vi "testArea.vi"() -> ()   [LabVIEW 2019]
panel:
  out "output array":dbl[](array[numeric])
  out "Area":dbl
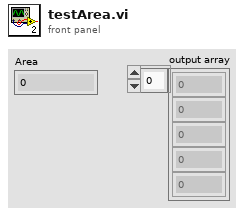
[diagram p1: front panel]
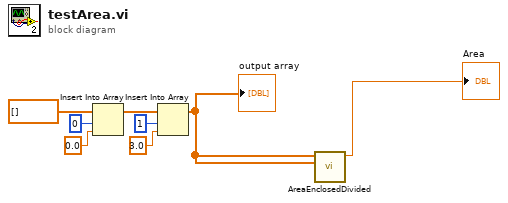
[diagram p0: block diagram]
diagram:
  n1 = Insert Into Array(array=dbl[] [], index=0, new element=0.0 ("new element/subarray")) -> (w3:dbl[])
  n2 = Insert Into Array(array=w3, index=1, new element=3.0 ("new element/subarray")) -> (w2:dbl[])
  "output array" <- w2
  n3 = call "AreaEnclosedDivided.vi"("H"=w2, "B"=w2) -> ("Area"=→"Area":dbl)  [unwired: 9 in]
